vi "Read Math Result.vi"(7 "Math Data Size (0)":i32, 8 "error in (no error)":errorcluster, 9 "Math Data Offset (0)":i32, 10 "Channel (1: Channel 1)":i32(ring)=1 items=["Channel 1"=1, "Channel 2"=2], 11 "VISA resource name":refnum<visa-resource-name>) -> (0 "error out":errorcluster, 2 "Math Data":T1, 3 "VISA resource name out":refnum<visa-resource-name>)   [LabVIEW 2012, in "Keysight B2980 Series.lvlib"]
doc: "Returns the calculation result data."
uses:
  Keysight B2980 Series.lvlib
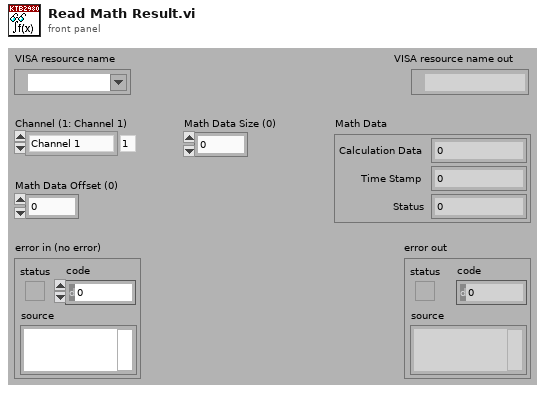
[diagram p1: front panel]
types:
  T1 = cluster{"Calculation Data":dbl, "Time Stamp":dbl, "Status":dbl}
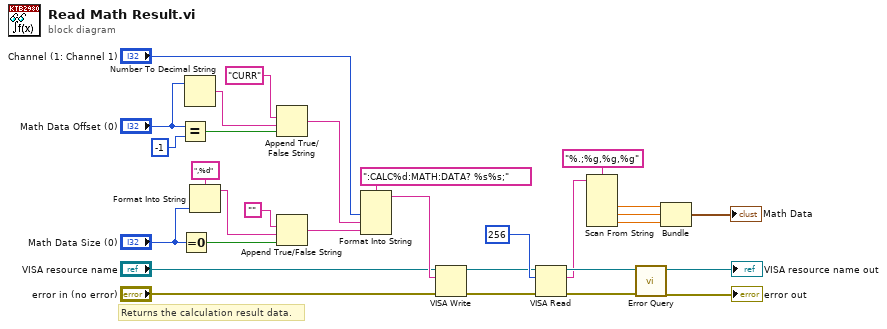
[diagram p0: block diagram]
diagram:
  # "Returns the calculation result data."
  n1 = Equal?(x="Math Data Offset (0)", y=-1) -> (x = y?=w6:bool)
  n2 = Equal To 0?(x="Math Data Size (0)") -> (x = 0?=w9:bool)
  n3 = Number To Decimal String(number="Math Data Offset (0)") -> (decimal integer string=w4:string)  [unwired: 1 out]
  n4 = Format Into String(format string=",%d", "Math Data Size (0)") -> (resulting string=w7:string)  [unwired: 2 in, 1 out]
  n5 = Append True/False String(1:w6, 2:w4, 3:"CURR") -> (0:w3:string)  [unwired: 1 in]
  n6 = Append True/False String(1:w9, 2:w7, 3:"") -> (0:w16:string)  [unwired: 1 in]
  n7 = Format Into String(format string=":CALC%d:MATH:DATA? %s%s;", "Channel (1: Channel 1)", w3, w16) -> (resulting string=w28:string)  [unwired: 2 in, 1 out]
  n8 = VISA Write(VISA resource name="VISA resource name", write buffer=w28, error in (no error)="error in (no error)") -> (VISA resource name out=w24:refnum<visa-resource-name>, error out=w23:errorcluster)  [unwired: 1 out]
  n9 = VISA Read(VISA resource name=w24, byte count=u32 256, error in (no error)=w23) -> (VISA resource name out=w22:refnum<visa-resource-name>, read buffer=w11:string, error out=w21:errorcluster)  [unwired: 1 out]
  n10 = Scan From String(format string="%.;%g,%g,%g", input string=w11) -> (output 1=w14:dbl, output 2=w13:dbl, output 3=w12:dbl)  [unwired: 2 in, 6 out]
  n11 = call "Error Query.vi"("error in (no error)"=w21, "VISA resource name"=w22) -> ("error out"=→"error out":errorcluster, "VISA resource name out"=→"VISA resource name out":refnum<visa-resource-name>)  [unwired: 8 out]
  n12 = Bundle(w14, w13, w12) -> (→"Math Data":cluster{dbl, dbl, dbl})  [unwired: 1 out]
